vi "AddAIDataSVtoLib.vi"(8 "error in (no error)":errorcluster, 10 "Name":string, 11 "Library in":refnum<vi>) -> (0 "error out":errorcluster, 3 "Library out":refnum<vi>)   [LabVIEW 2013]
uses:
  AI_Data.ctl
  NI Card.lvclass
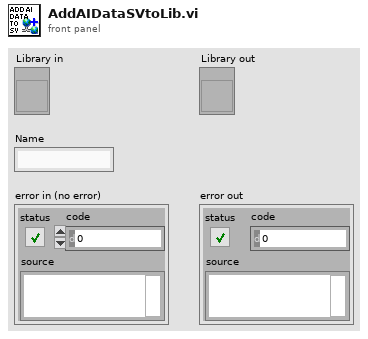
[diagram p1: front panel]
types:
  T1 = enum16{"Single-Process", "Network-Published", "Time-Triggered", "Industrial"}
  T2 = typedef "NI Card.lvclass/AI_Data.ctl" = cluster{"t":dbl[], "y":dbl[], "Channel Name":string}
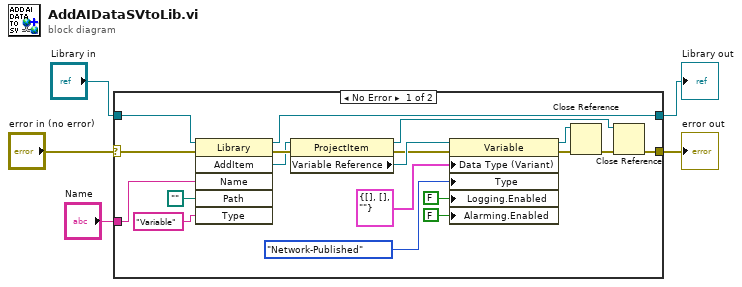
[diagram p0: block diagram]
diagram:
  n1 = case shown="No Error" "error in (no error)" {
    selector: "error in (no error)" -> [w6 w26]
    tunnel: "Name" -> [w24 _]
    tunnel: [w22 w26] -> w4
    tunnel: [w21 w25] -> w3
    tunnel: "Library in" -> [w20 w25]
    frame No Error {
      n2 = invoke class="Library" method="AddItem"(reference=w20, error in=w6, "Name"=w24, "Path"=path "", "Type"="Variable") -> (reference out=w21:refnum<vi>, error out=w23:errorcluster, "AddItem"=w12:refnum<vi>)  [unwired: 1 in, 3 out]
      n3 = property class="ProjectItem"(reference=w12, error in=w23) -> (reference out=w19:refnum<vi>, error out=w8:errorcluster, "Variable Reference"=w11:refnum<vi>)
      n4 = property class="Variable"(reference=w11, error in=w8, "Data Type (Variant)"=T2 {"t"=[], "y"=[], "Channel Name"=""} ("AI Data"), "Type"=T1."Network-Published", "Logging.Enabled"=FALSE ("Logging:Enabled"), "Alarming.Enabled"=FALSE ("Alarming:Enabled")) -> (reference out=w18:refnum<vi>, error out=w17:errorcluster)
      n5 = Close Reference(reference=w18, error in (no error)=w17) -> (error out=w16:errorcluster)
      n6 = Close Reference(reference=w19, error in (no error)=w16) -> (error out=w22:errorcluster)
    }
    frame Error {
    }
  }
  "error out" <- w4
  "Library out" <- w3
